vi "LVFunction_Imop_GetHasoSerialNumberFromConfigFile.vi"(0 "Configuration file path":path, 11 "error in":errorcluster) -> (4 "HasoSerialNumber":string, 15 "error out":errorcluster)   [LabVIEW 2018]
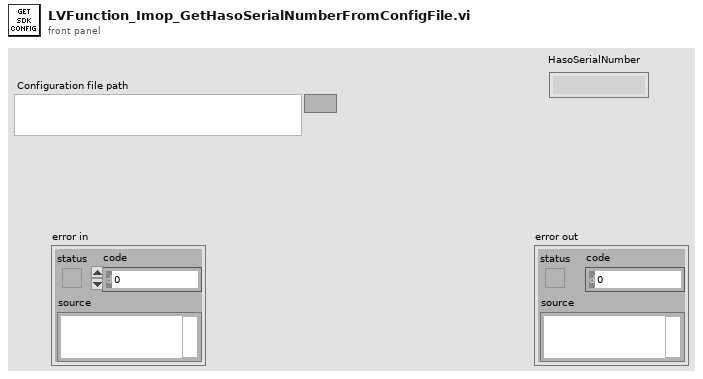
[diagram p1: front panel]
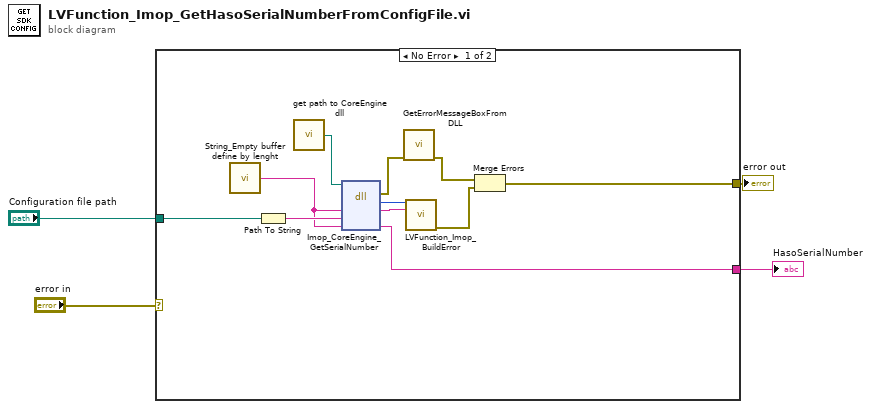
[diagram p0: block diagram]
diagram:
  n1 = case shown="No Error" "error in" {
    selector: "error in" -> [_ w16]
    tunnel: [w9 w16] -> w3
    tunnel: "Configuration file path" -> [w8 _]
    tunnel: [w5 _] -> w1
    frame No Error {
      n2 = call "String_Empty buffer define by lenght.vi"() -> ("Empty buffer"=w6:string)  [unwired: 1 in]
      n3 = Path To String(path=w8) -> (string=w7:string)
      n4 = call "get path to CoreEngine dll.vi"() -> ("path to wavekit library"=w12:path)  [unwired: 14 in, 1 out]
      n5 = dll-call lib="D:/soft/HASO_v3/SVN_trunk/ImOpCoreEngine4_LV2011/DLLs/c_interface_vc100.dll" fn="Imop_CoreEngine_GetSerialNumber"(path in=w12, "message"=w6, "config_file_path"=w7, "HasoSerialNumber"=w6) -> (error out=w13:errorcluster, "return type"=w11:i32, "message"=w10:string, "HasoSerialNumber"=w5:string)  [unwired: 3 in, 1 out]
      n6 = call "GetErrorMessageBoxFromDLL.vi"("error IN"=w13) -> ("error OUT"=w14:errorcluster)  [unwired: 10 in]
      n7 = call "LVFunction_Imop_BuildError.vi"("code"=w11, "String to Prepend to source (\"\")"=w10) -> ("error out"=w15:errorcluster)  [unwired: 13 in]
      n8 = Merge Errors(w14, w15) -> (w9:errorcluster)
    }
    frame Error {
    }
  }
  "error out" <- w3
  "HasoSerialNumber" <- w1
